vi "Stage1.vi"(8 "Obs Distances Measure Array":dbl[](array[numeric]), 9 "Posture In":dbl[](array[numeric]), 10 "Robot Frame (World)":cluster{"X":sgl, "Y":sgl, "Theta":dbl}, 11 "Start":bool=TRUE) -> (1 "Frame Velocity":dbl[](array[numeric]), 2 "Finish Stage?":bool=TRUE, 3 "Current State":string="Next Goal")   [LabVIEW 2016]
uses:
  MainStateControl.ctl
  WaitVI/Wait Command.ctl
panel:
  out "output cluster":T2
  in  "Init Cluster":T2={"Current State"=enum."Start", "Next Goal"={"X"=0.0, "Y"=0.0, "theta"=0.0}, "Goal Index"=0}
  in  "Goal list":cluster{"X":sgl, "Y":sgl, "theta":dbl}[](array[cluster])=[{"X"=-0.75, "Y"=1.4, "theta"=1.57}, {"X"=-0.1, "Y"=3.5, "theta"=0.0}, {"X"=0.0, "Y"=0.0, "theta"=0.0}]
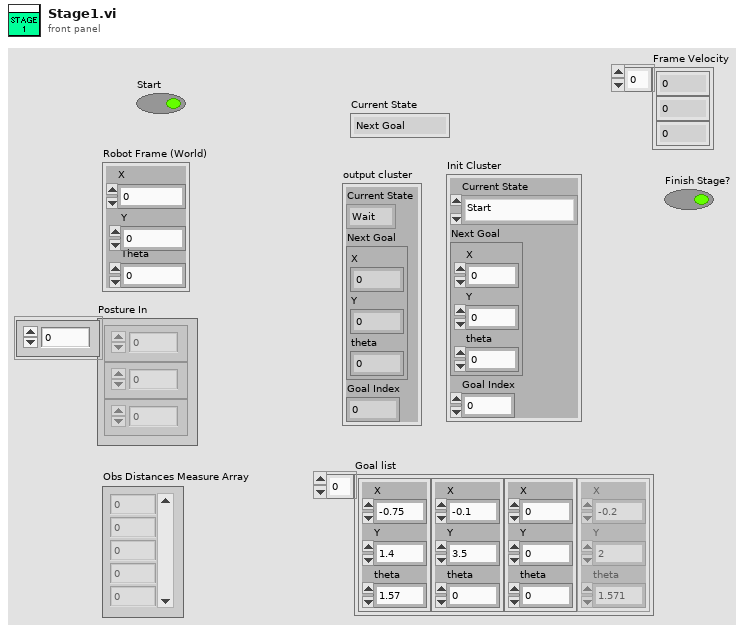
[diagram p1: front panel]
types:
  T1 = typedef "MainStateControl.ctl" = enum16{"Wait", "Next Goal", "Driving", "Start", "Stop"}
  T2 = cluster{"Current State":T1, "Next Goal":cluster{"X":sgl, "Y":sgl, "theta":dbl}, "Goal Index":i32}
  T3 = typedef "Wait Command.ctl" = enum16{"Running", "Init"}
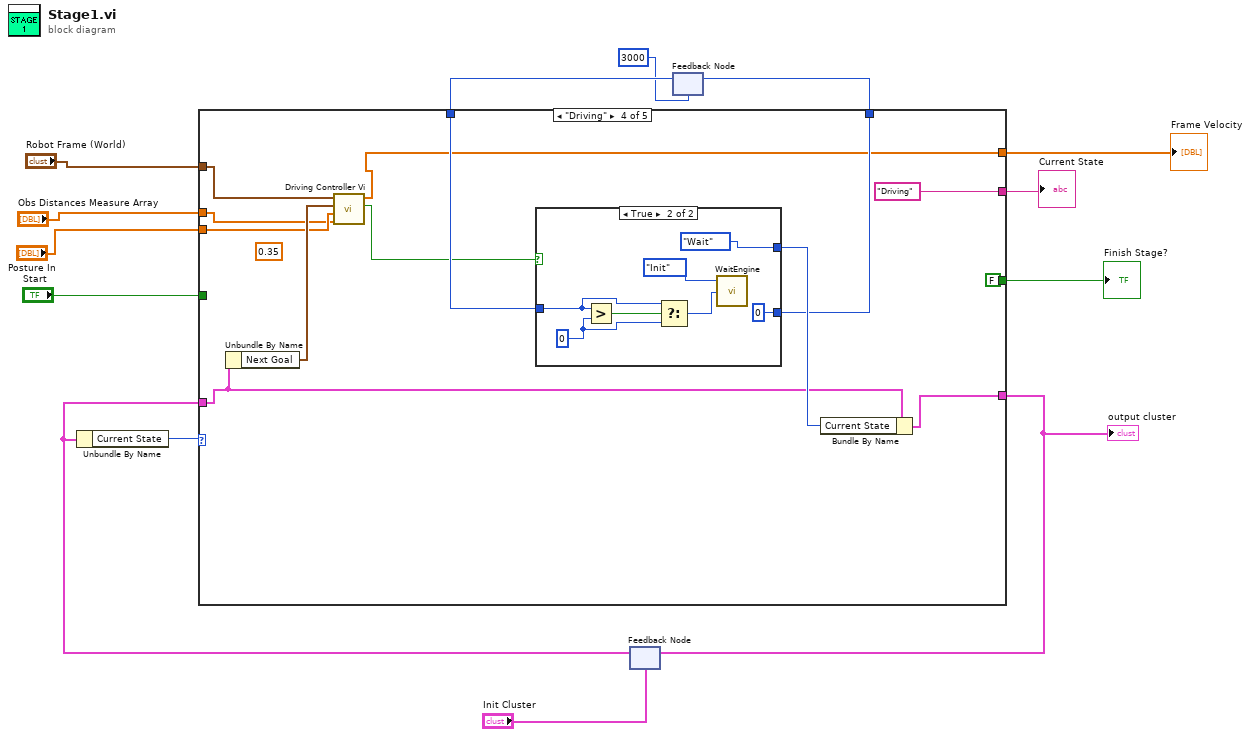
[diagram p0: block diagram]
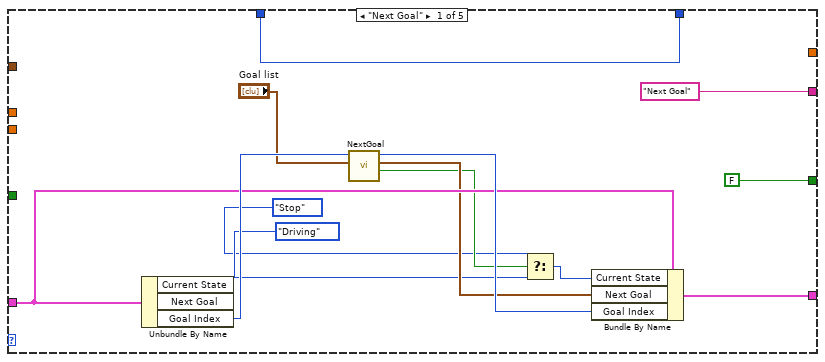
[diagram p2: hidden frame]
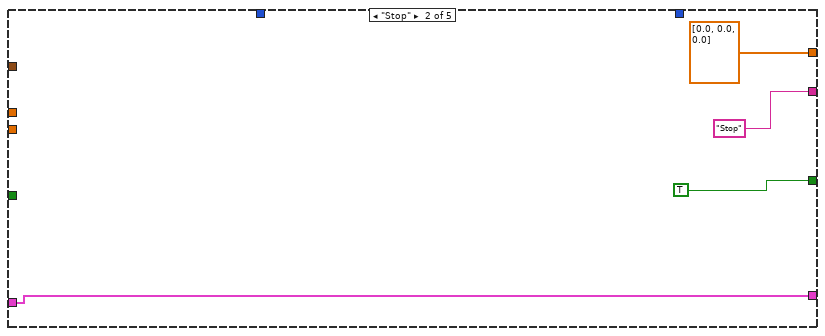
[diagram p3: hidden frame]
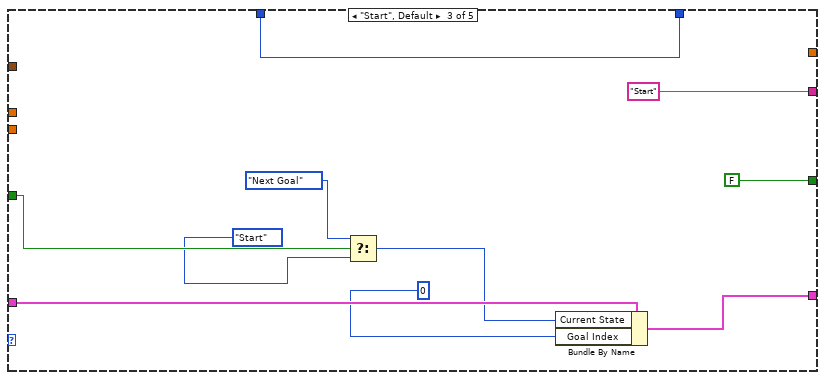
[diagram p4: hidden frame]
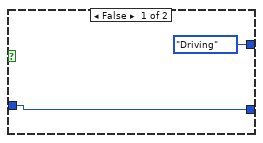
[diagram p5: hidden frame]
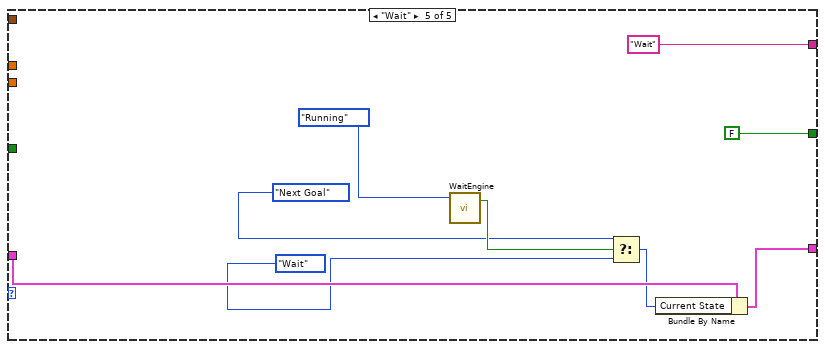
[diagram p6: hidden frame]
diagram:
  n1 = feedback #1("Init Cluster") -> (w10:T2)
  n2 = Unbundle By Name(w10) -> ("Current State"=w11:T1)
  n3 = feedback #2(u32 3000 ("Wait Time (ms)")) -> (w2:u32)
  n4 = case shown="\"Driving\"" w11 {
    tunnel: "Start" -> [_ _ w41 _ _]
    tunnel: ["Next Goal" "Stop" "Start" "Driving" "Wait"] -> w13
    tunnel: w10 -> [w24 w31 w38 w50 w70]
    tunnel: [w22 w31 w37 w54 w69] -> w9
    tunnel: [FALSE TRUE FALSE FALSE FALSE] -> w8
    tunnel: "Robot Frame (World)" -> [_ _ _ w47 _]
    tunnel: [_ dbl[] [0.0, 0.0, 0.0] ("Frame Velocity") _ w43 _] -> w6
    tunnel: "Obs Distances Measure Array" -> [_ _ _ w44 _]
    tunnel: "Posture In" -> [_ _ _ w45 _]
    tunnel: [w15 _ w32 w49 _] -> w3
    tunnel: w2 -> [w15 _ w32 w48 _]
    frame "Next Goal" {
      n5 = Unbundle By Name(w24) -> ("Goal Index"=w26:i32)  [unwired: 2 out]
      n6 = call "NextGoal.vi"("Goal list"="Goal list", "Current Index"=w26) -> ("Finish track?"=w21:bool, "Next Goal"=w23:cluster{"X":sgl, "Y":sgl, "theta":dbl}, "Goal Index"=w25:i32)  [unwired: 7 in]
      n7 = Select(t=MainStateControl."Stop" ("Enum"), s=w21, f=MainStateControl."Driving" ("Enum")) -> (s? t:f=w19:T1)
      n8 = Bundle By Name(cluster=w24, "Current State"=w19, "Next Goal"=w23, "Goal Index"=w25) -> (w22:T2)
    }
    frame "Stop" {
    }
    frame "Start", Default {
      n9 = Select(t=MainStateControl."Next Goal", s=w41, f=MainStateControl."Start") -> (s? t:f=w36:T1)
      n10 = Bundle By Name(cluster=w38, "Current State"=w36, "Goal Index"=0) -> (w37:T2)
    }
    frame "Driving" {
      (unwired) 0.35 ("V Forward")
      n11 = Unbundle By Name(w50) -> ("Next Goal"=w46:cluster{"X":sgl, "Y":sgl, "theta":dbl})
      n12 = call "Driving Controller Vi.vi"("Obs Distances Measure Array"=w44, "Posture In"=w45, "Goal Frame (World)"=w46, "Robot Frame (World)"=w47) -> ("Goal Arrived?"=w42:bool, "Frame Velocity"=w43:dbl[])  [unwired: 6 in]
      n13 = case shown="True" w42 {
        tunnel: [MainStateControl."Driving" ("Enum") MainStateControl."Wait" ("Enum")] -> w52
        tunnel: w48 -> [w55 w60]
        tunnel: [w55 u32 0 ("Wait Time (ms)")] -> w49
        frame False {
        }
        frame True {
          w59 = u32 0 ("y")
          n14 = Greater?(x=w60, y=w59) -> (0:w61:bool)
          n15 = Select(t=w60, s=w61, f=w59) -> (s? t:f=w58:u32)
          n16 = call "WaitEngine.vi"("Wait Time (ms)"=w58, "Wait Command"=Wait_Command."Init") -> ()  [unwired: 2 in, 1 out]
        }
      }
      n17 = Bundle By Name(cluster=w50, "Current State"=w52) -> (w54:T2)
    }
    frame "Wait" {
      n18 = call "WaitEngine.vi"("Wait Command"=Wait_Command."Running") -> ("Elapsed?"=w71:bool)  [unwired: 3 in]
      n19 = Select(t=MainStateControl."Next Goal" ("Enum"), s=w71, f=MainStateControl."Wait" ("Enum")) -> (s? t:f=w67:T1)
      n20 = Bundle By Name(cluster=w70, "Current State"=w67) -> (w69:T2)
    }
  }
  "Current State" <- w13
  "output cluster" <- w9
  "Finish Stage?" <- w8
  "Frame Velocity" <- w6
  n21 = feedback-in #1(w9) -> ()
  n22 = feedback-in #2(w3) -> ()
